vi "Create (with Extension).vi"(8 "error in (no error)":errorcluster, 11 "Image File Extension":string(combo)=".bmp") -> (0 "error out":errorcluster, 3 "Image to File-Buffer Encoder":refnum<class "Image to File-Buffer Encoder.lvclass">)   [LabVIEW 2020, in "image.lvlib" / "Image to File-Buffer Encoder.lvclass"]
uses:
  Image to File-Buffer Encoder.lvclass
  Image to File-Buffer Encoder.lvclass/Image to File-Buffer Encoder.ctl
  1ced6358-dfcc-4e78-9c26-089d6408b6c9.vi
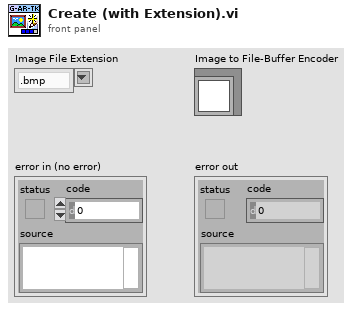
[diagram p1: front panel]
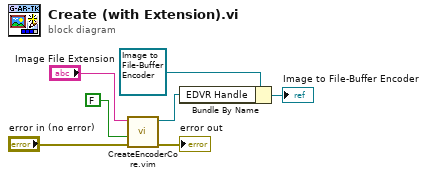
[diagram p0: block diagram]
diagram:
  n1 = call "CreateEncoderCore.vim"("error in (no error)"="error in (no error)", "SaveAlpha"=FALSE, "Extension"="Image File Extension") -> ("error out"=→"error out":errorcluster, "EDVR Handle"=w5:refnum<data-value>)  [unwired: 7 in]
  n2 = Bundle By Name(cluster=refnum<class "Image to File-Buffer Encoder.lvclass"> refnum ("Image to File-Buffer Encoder out"), "EDVR Handle"=w5) -> (→"Image to File-Buffer Encoder":refnum<class "Image to File-Buffer Encoder.lvclass">)
